vi "Control Transmit.vi"(8 "error in (no error)":errorcluster, 11 "Sensor General Class in":refnum<class "Sensor General Class.lvclass">) -> (0 "error out":errorcluster, 3 "Sensor General Class out":refnum<class "Sensor General Class.lvclass">)   [LabVIEW 2020, in "Sensor General Class.lvclass"]
uses:
  Sensor General Class.lvclass
  Sensor General Class.lvclass/Sensor General Class.ctl
  <vilib>/Utility/error.llb/Error Cluster From Error Code.vi
  <vilib>/ErrorRing/Error Ring.xnode
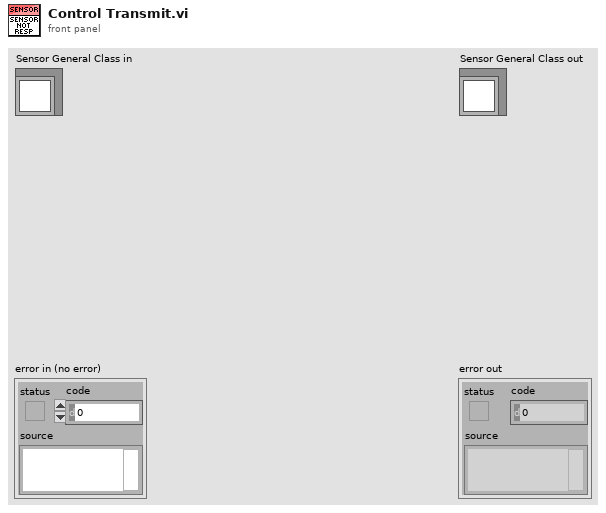
[diagram p1: front panel]
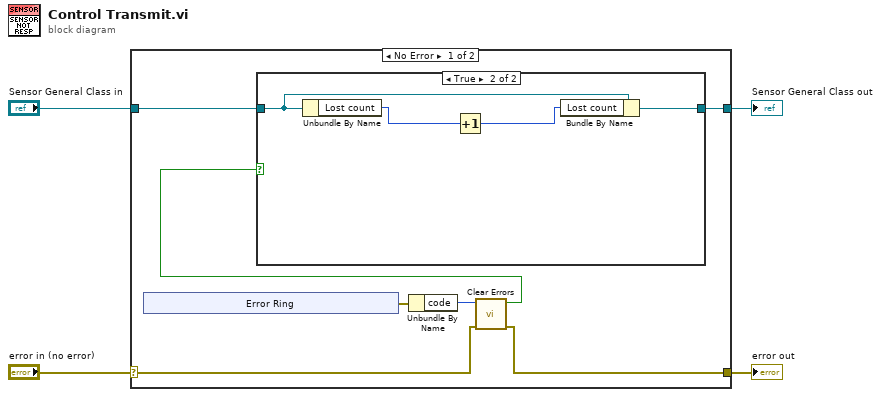
[diagram p0: block diagram]
diagram:
  n1 = case shown="No Error" "error in (no error)" {
    selector: "error in (no error)" -> [w9 w22]
    tunnel: [w8 w22] -> w3
    tunnel: [w5 w21] -> w1
    tunnel: "Sensor General Class in" -> [w7 w21]
    frame No Error {
      n2 = xnode "Error Ring"() -> ("error out"=w11:errorcluster)
      n3 = Unbundle By Name(w11) -> ("code"=w10:i32)
      n4 = call <vilib>:"Clear Errors.vi"("error in (no error)"=w9, "specific error code to clear (0: all)"=w10) -> ("error out"=w8:errorcluster, "specific error cleared?"=w6:bool)  [unwired: 4 in]
      n5 = case shown="True" w6 {
        tunnel: w7 -> [w12 w16]
        tunnel: [w12 w15] -> w5
        frame False {
        }
        frame True {
          n6 = Unbundle By Name(w16) -> ("Lost count"=w14:i32)
          n7 = Increment(x=w14) -> (x+1=w13:i32)
          n8 = Bundle By Name(cluster=w16, "Lost count"=w13) -> (w15:refnum<class "Sensor General Class.lvclass">)
        }
      }
    }
    frame Error {
    }
  }
  "error out" <- w3
  "Sensor General Class out" <- w1
